vi "get_attributes.vi"(8 "error in (no error)":errorcluster caption="entrée d'erreur (pas d'erreur)", 11 "LinearDiscriminantAnalysis.lvclass 2":refnum<class "LinearDiscriminantAnalysis.lvclass">) -> (0 "error out":errorcluster caption="sortie d'erreur", 3 "LinearDiscriminantAnalysis.lvclass":refnum<class "LinearDiscriminantAnalysis.lvclass">)   [LabVIEW 2020, in "LinearDiscriminantAnalysis.lvclass"]
uses:
  LinearDiscriminantAnalysis.lvclass
  LinearDiscriminantAnalysis.lvclass/LinearDiscriminantAnalysis.ctl
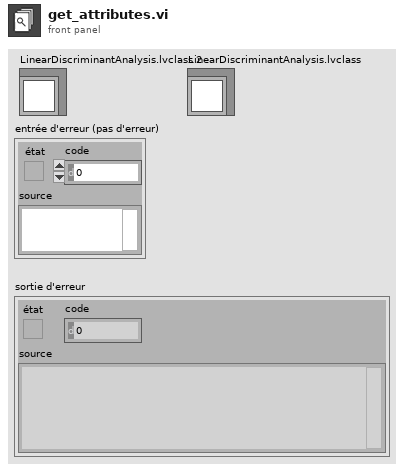
[diagram p1: front panel]
types:
  T1 = typedef "linear_discriminant_analysis_attributes.ctl" = cluster{"coef_":dbl[][], "intercept_":dbl[], "covariance_":dbl[][], "explained_variance_ratio_":dbl[], "means_":dbl[][], "priors_":dbl[], "scalings_":dbl[][], "xbar_":dbl[], "classes_":dbl[]}
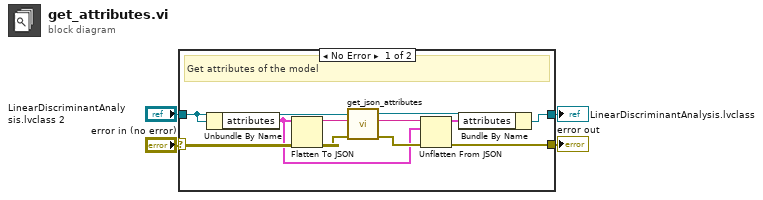
[diagram p0: block diagram]
diagram:
  n1 = case shown="No Error" "error in (no error)" {
    selector: "error in (no error)" -> [w13 w17]
    tunnel: [w5 w17] -> w3
    tunnel: "LinearDiscriminantAnalysis.lvclass 2" -> [w10 w16]
    tunnel: [w6 w16] -> w1
    frame No Error {
      # "Get attributes of the model"
      n2 = Unbundle By Name(w10) -> ("attributes"=w9:T1)
      n3 = Flatten To JSON(anything=w9, error in (no error)=w13) -> (JSON string=w12:string, 11:w11:errorcluster)  [unwired: 1 in]
      n4 = call-dynamic "get_json_attributes.vi"("error in (no error)"=w11, "format"=w12, "Model en entrée"=w10) -> ("error out"=w14:errorcluster, "valeur renvoyée"=w15:string, "Model en sortie"=w8:refnum<class "LinearDiscriminantAnalysis.lvclass">)  [unwired: 6 in]
      n5 = Unflatten From JSON(JSON string=w15, type and defaults=w9, error in (no error)=w14) -> (value=w7:T1, error out=w5:errorcluster)  [unwired: 4 in]
      n6 = Bundle By Name(cluster=w8, "attributes"=w7) -> (w6:refnum<class "LinearDiscriminantAnalysis.lvclass">)
    }
    frame Error {
    }
  }
  "error out" <- w3
  "LinearDiscriminantAnalysis.lvclass" <- w1
